vi "zadanie 2.vi"() -> ()   [LabVIEW 2013]
panel:
  out "initialized array":dbl[](array[numeric])
  in  "Numeric":dbl
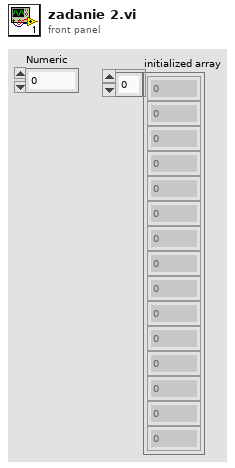
[diagram p1: front panel]
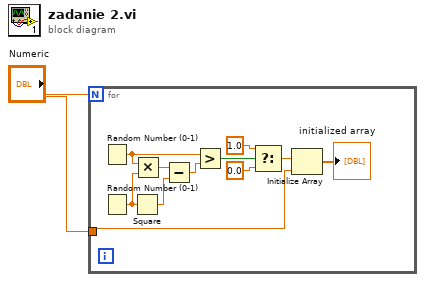
[diagram p0: block diagram]
diagram:
  n1 = for {
    N: "Numeric" -> [_]
    tunnel: "Numeric" -> [w10]
    n2 = Random Number (0-1)() -> (number: 0 to 1=w3:dbl)
    n3 = Random Number (0-1)() -> (number: 0 to 1=w7:dbl)
    n4 = Square(x=w7) -> (x^2=w6:dbl)
    n5 = Multiply(x=w3, y=w7) -> (x*y=w5:dbl)
    n6 = Subtract(x=w5, y=w6) -> (x-y=w4:dbl)
    n7 = Greater?(x=w3, y=w4) -> (0:w2:bool)
    n8 = Select(t=1.0, s=w2, f=0.0) -> (s? t:f=w9:dbl)
    n9 = Initialize Array(w9, w10) -> (→"initialized array":dbl[])
  }
